vi "initialize.vi"(8 "error in (no error)":errorcluster, 9 "qeue name":string, 10 "remote IP":string, 11 "Server in":refnum<class "Server.lvclass">) -> (0 "error out":errorcluster, 3 "Server out":refnum<class "Server.lvclass">)   [LabVIEW 2018, in "Server.lvclass"]
uses:
  Server.lvclass
  Server.lvclass/Server.ctl
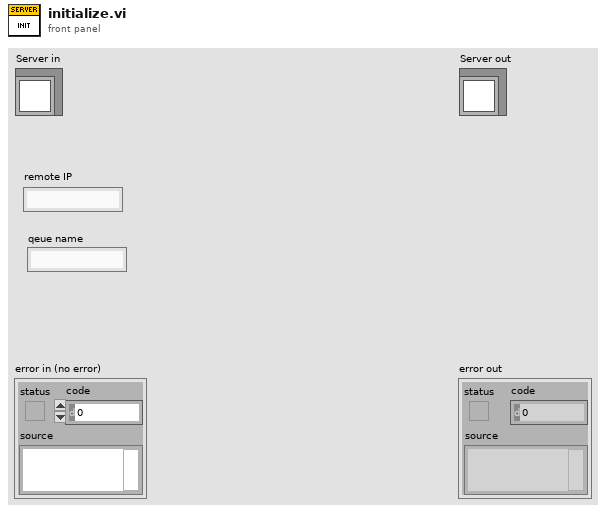
[diagram p1: front panel]
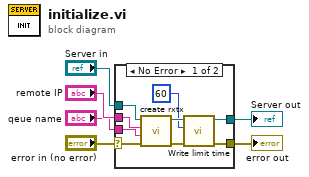
[diagram p0: block diagram]
diagram:
  n1 = case shown="No Error" "error in (no error)" {
    selector: "error in (no error)" -> [w15 w17]
    tunnel: [w13 w17] -> w5
    tunnel: [w11 w16] -> w3
    tunnel: "Server in" -> [w10 w16]
    tunnel: "remote IP" -> [w8 _]
    tunnel: "qeue name" -> [w7 _]
    frame No Error {
      n2 = call "create rxtx.vi"("error in (no error)"=w15, "qeue name"=w7, "remote IP"=w8, "Server in"=w10) -> ("error out"=w14:errorcluster, "Server out"=w12:refnum<class "Server.lvclass">)  [unwired: 6 in]
      n3 = call "Write limit time.vi"("error in (no error)"=w14, "limit time"=u16 60, "Server in"=w12) -> ("error out"=w13:errorcluster, "Server out"=w11:refnum<class "Server.lvclass">)  [unwired: 7 in]
    }
    frame Error {
    }
  }
  "error out" <- w5
  "Server out" <- w3
